vi "Write Phone Number.vi"(8 "error in (no error)":errorcluster, 10 "Phone Number":string, 11 "Phone Number in":refnum<class "Phone Number.lvclass">) -> (0 "error out":errorcluster, 3 "Phone Number out":refnum<class "Phone Number.lvclass">)   [LabVIEW 2015, in "NI_AWS_SNS.lvlib" / "Phone Number.lvclass"]
uses:
  Phone Number.lvclass
  Phone Number.lvclass/Phone Number.ctl
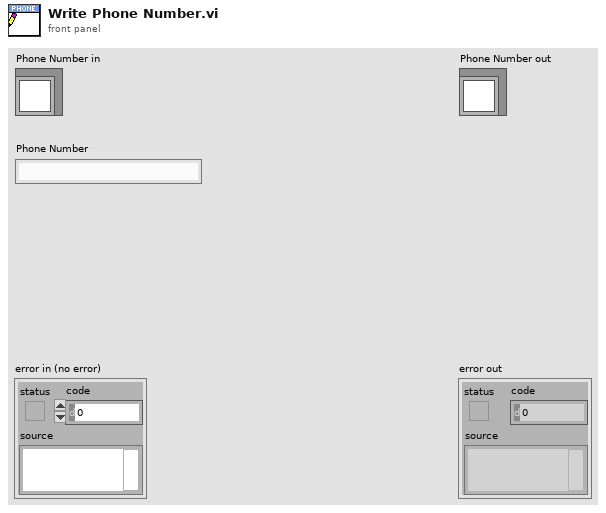
[diagram p1: front panel]
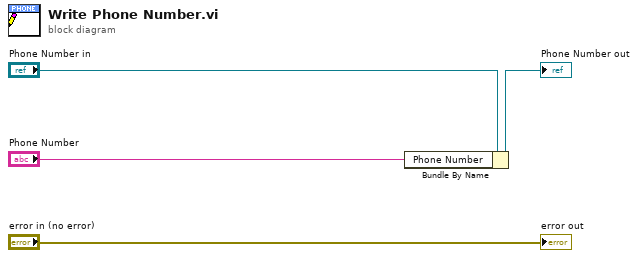
[diagram p0: block diagram]
diagram:
  n1 = Bundle By Name(cluster="Phone Number in", "Phone Number"="Phone Number") -> (→"Phone Number out":refnum<class "Phone Number.lvclass">)
  "error out" <- "error in (no error)"
